vi "SlowNearWaypoint.vi"(3 "Current Lon.":dbl, 4 "Current Lat.":dbl, 5 "Waypoint Lon.":dbl, 6 "Waypoint Lat.":dbl) -> (0 "SpeedDecrease":dbl)   [LabVIEW 2010]
doc: "This VI checks to see if the robots curretn position is close to the next waypoint. If it is, it sets a boolean flag to allow a case statement to slow down robot"
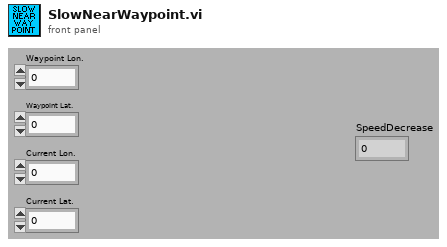
[diagram p1: front panel]
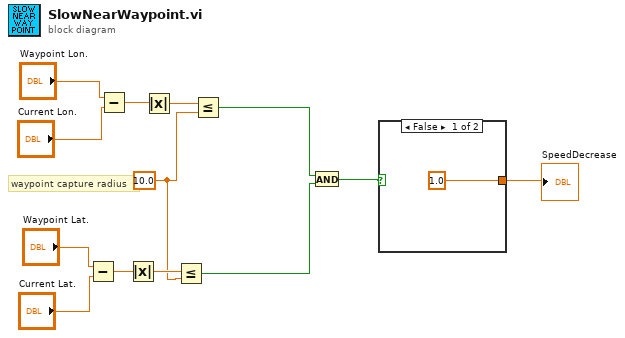
[diagram p0: block diagram]
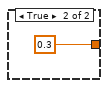
[diagram p2: hidden frame]
diagram:
  w5 = 10.0 ("y")
  # "waypoint capture radius"
  n1 = Subtract(x="Waypoint Lat.", y="Current Lat.") -> (x-y=w8:dbl)
  n2 = Subtract(x="Waypoint Lon.", y="Current Lon.") -> (x-y=w9:dbl)
  n3 = Absolute Value(x=w8) -> (abs(x)=w7:dbl)
  n4 = Absolute Value(x=w9) -> (abs(x)=w6:dbl)
  n5 = Less Or Equal?(x=w7, y=w5) -> (x <= y?=w3:bool)
  n6 = Less Or Equal?(x=w6, y=w5) -> (x <= y?=w4:bool)
  n7 = And(x=w4, y=w3) -> (x .and. y?=w1:bool)
  n8 = case shown="False" w1 {
    tunnel: [1.0 0.3] -> w2
    frame False {
    }
    frame True {
    }
  }
  "SpeedDecrease" <- w2
